vi "test_connection_example.vi"() -> ()   [LabVIEW 2017]
panel:
  out "Numeric 3":dbl
  in  "stop":bool
  in  "Slide 3":dbl(slide) scale=0.0..10.0
  in  "Slide 2":dbl(slide) scale=0.0..10.0
  in  "Slide":dbl(slide) scale=0.0..10.0
  out "Numeric 2":dbl
  in  "Numeric":dbl
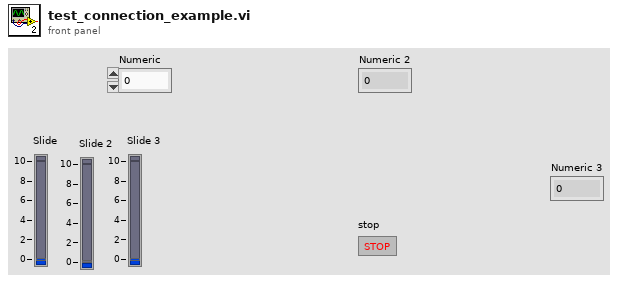
[diagram p1: front panel]
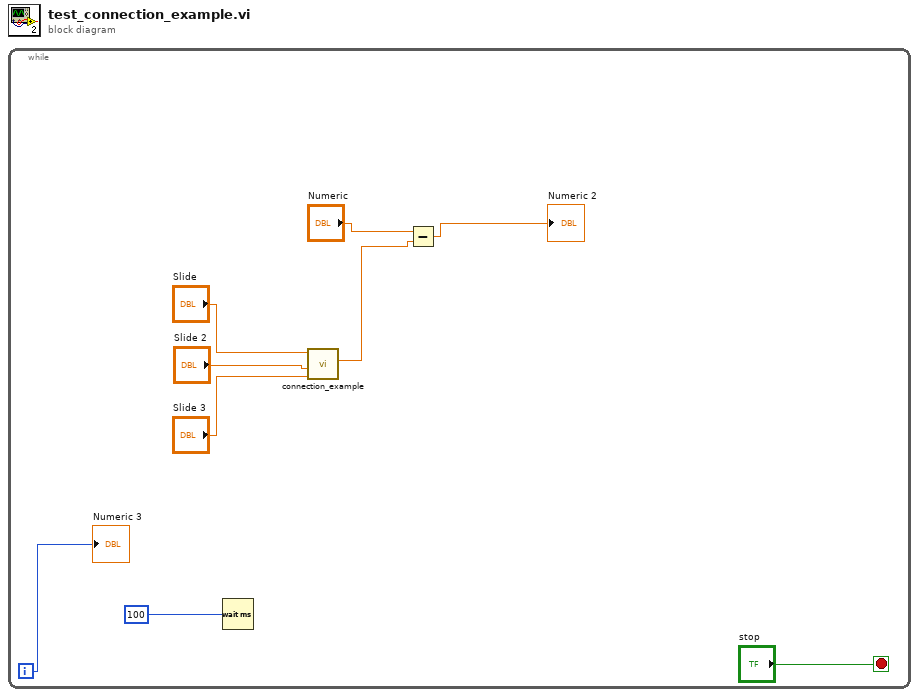
[diagram p0: block diagram]
diagram:
  n1 = while {
    i -> [w1]
    stop <- "stop" stop-if-true
    n2 = Wait (ms)(milliseconds to wait=u32 100) -> ()  [unwired: 1 out]
    n3 = call "connection_example.vi"("Numeric 3"="Slide 3", "Numeric 2"="Slide 2", "Numeric"="Slide") -> ("Numeric 4"=w7:dbl)
    n4 = Subtract(x="Numeric", y=w7) -> (x-y=→"Numeric 2":dbl)
    "Numeric 3" <- w1
  }
